vi "User Interface.vi"(8 "error in (no error)":errorcluster, 11 "User Interface in":refnum<class "User Interface.lvclass">) -> (0 "error out":errorcluster, 3 "User Interface out":refnum<class "User Interface.lvclass">)   [LabVIEW 2017, in "DSF Core.lvlib" / "Core Channel User Interface.lvclass"]
uses:
  Core Channel User Interface.lvclass
  User Interface.lvclass
  Configuration/Configuration.lvclass
  Configuration/Base/Channel/Channel Configuration.lvclass
  C:/Git/DSF/Core/Classes/Configuration/Configuration.lvclass
panel:
  out "Data Version":string
  in  "String Data Type":T1(ring)
  in  "Engine Data Type":T1(ring)
  in  "String Offset":u64 format="%d bytes"
  in  "Units":string
  in  "Name":string
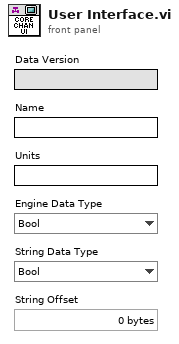
[diagram p1: front panel]
types:
  T1 = enum8{"Bool", "SGL", "DBL", "I8", "I16", "I32", "I64", "U8", "U16", "U32", "U64"}
  T2 = typedef "DSF Core.lvlib/DSF Core Channel Configuration.ctl" = cluster{"name":string, "units":string, "engine data type":T3, "string data type":T3, "string offset":u64}
  T3 = typedef "DSF Core.lvlib/DSF Data Type.ctl" = enum8{"Bool", "SGL", "DBL", "I8", "I16", "I32", "I64", "U8", "U16", "U32", "U64"}
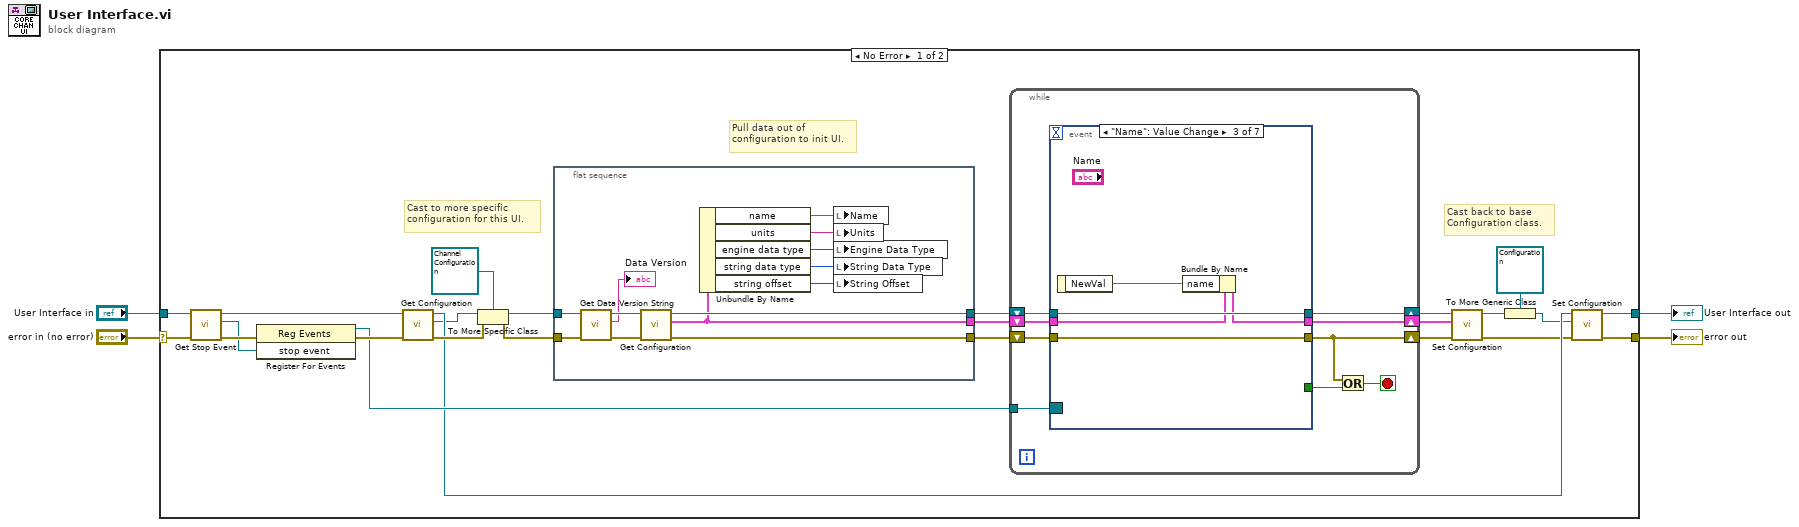
[diagram p0: block diagram]
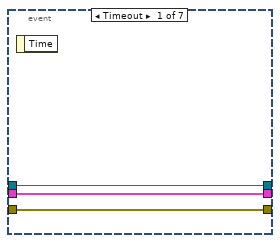
[diagram p2: hidden frame]
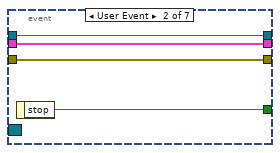
[diagram p3: hidden frame]
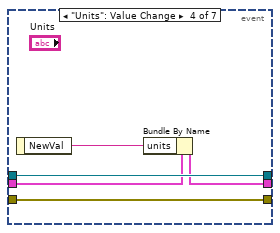
[diagram p4: hidden frame]
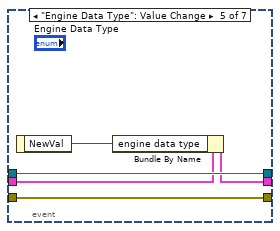
[diagram p5: hidden frame]
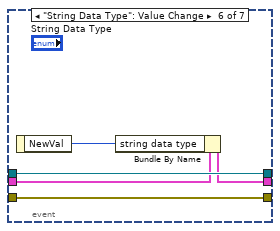
[diagram p6: hidden frame]
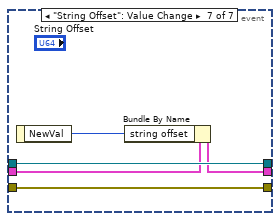
[diagram p7: hidden frame]
diagram:
  n1 = case shown="No Error" "error in (no error)" {
    selector: "error in (no error)" -> [w21 w85]
    tunnel: "User Interface in" -> [w20 w84]
    tunnel: [w14 w84] -> w1
    tunnel: [w15 w85] -> w3
    frame No Error {
      # "Pull data out of configuration to init UI."
      # "Cast back to base Configuration class."
      # "Cast to more specific configuration for this UI."
      n2 = call "Get Stop Event.vi"("error in (no error)"=w21, "User Interface in"=w20) -> ("error out"=w19:errorcluster, "stop event"=w18:refnum<user-event>, "User Interface out"=w17:refnum<class "User Interface.lvclass">)  [unwired: 7 in]
      n3 = register-events(error in=w19, w18) -> (reference out=w16:refnum<event-registration>, error out=w23:errorcluster)  [unwired: 1 in]
      n4 = call "Get Configuration.vi"("error in (no error)"=w23, "User Interface in"=w17) -> ("error out"=w22:errorcluster, "configuration"=w12:refnum<class "Configuration.lvclass">, "User Interface out"=w13:refnum<class "User Interface.lvclass">)  [unwired: 7 in]
      n5 = To More Specific Class(target class=refnum<class "Channel Configuration.lvclass"> refnum ("DSF Core.lvlib:Channel Configuration.lvclass"), reference=w12, error in=w22) -> (specific class reference=w27:refnum<class "Channel Configuration.lvclass">, error out=w28:errorcluster)
      n6 = flat-sequence {
        tunnel: [w32] -> w25
        tunnel: w28 -> [w36]
        tunnel: w27 -> [w37]
        tunnel: [w33] -> w26
        tunnel: [w31] -> w24
        frame #0 {
          n7 = call "Get Data Version String.vi"("error in (no error)"=w36, "Configuration in"=w37) -> ("error out"=w34:errorcluster, "data version"=→"Data Version":string, "Configuration out"=w35:refnum<class "Channel Configuration.lvclass">)  [unwired: 7 in]
          n8 = call "Get Configuration.vi"("error in (no error)"=w34, "Core Channel Configuration in"=w35) -> ("error out"=w32:errorcluster, "configuration"=w31:T2, "Core Channel Configuration out"=w33:refnum<class "Channel Configuration.lvclass">)  [unwired: 7 in]
          n9 = Unbundle By Name(w31) -> ("name"=w42:string, "units"=w41:string, "engine data type"=w40:T3, "string data type"=w39:T3, "string offset"=w38:u64)
          n10 = local write "Name"(w42) -> ()
          n11 = local write "Units"(w41) -> ()
          n12 = local write "Engine Data Type"(w40) -> ()
          n13 = local write "String Data Type"(w39) -> ()
          n14 = local write "String Offset"(w38) -> ()
        }
      }
      n15 = while {
        tunnel: w16 -> [w51]
        shift-right: [w49] -> w9
        shift-left: w25 -> [w50]
        shift-right: [w45] -> w7
        shift-left: w26 -> [w46]
        shift-right: [w43] -> w5
        shift-left: w24 -> [w44]
        stop <- w48 stop-if-true
        n16 = event shown="[2] \"Name\": Value Change" {
          selector: w51 -> [_ _ _ _ _ _ _]
          dyn-events: _ -> [_ _ _ _ _ _ _]
          timeout: _ -> [_ _ _ _ _ _ _]
          tunnel: [_ w56 _ _ _ _ _] -> w47
          tunnel: w50 -> [w54 w58 w62 w67 w72 w77 w82]
          tunnel: [w54 w58 w62 w67 w72 w77 w82] -> w49
          tunnel: w46 -> [w53 w57 w63 w68 w73 w78 w83]
          tunnel: [w53 w57 w63 w68 w73 w78 w83] -> w45
          tunnel: w44 -> [w52 w55 w60 w65 w70 w75 w80]
          tunnel: [w52 w55 w59 w64 w69 w74 w79] -> w43
          event Timeout {
            n17 = event-data() -> ()  [unwired: 1 in, 1 out]
          }
          event User Event {
            n18 = event-data() -> ("stop"=w56:bool)  [unwired: 1 in]
          }
          event "Name": Value Change {
            n19 = event-data() -> ("NewVal"=w61:string)  [unwired: 1 in]
            n20 = Bundle By Name(cluster=w60, "name"=w61) -> (w59:T2)
          }
          event "Units": Value Change {
            n21 = event-data() -> ("NewVal"=w66:string)  [unwired: 1 in]
            n22 = Bundle By Name(cluster=w65, "units"=w66) -> (w64:T2)
          }
          event "Engine Data Type": Value Change {
            n23 = event-data() -> ("NewVal"=w71:T1)  [unwired: 1 in]
            n24 = Bundle By Name(cluster=w70, "engine data type"=w71) -> (w69:T2)
          }
          event "String Data Type": Value Change {
            n25 = event-data() -> ("NewVal"=w76:T1)  [unwired: 1 in]
            n26 = Bundle By Name(cluster=w75, "string data type"=w76) -> (w74:T2)
          }
          event "String Offset": Value Change {
            n27 = event-data() -> ("NewVal"=w81:u64)  [unwired: 1 in]
            n28 = Bundle By Name(cluster=w80, "string offset"=w81) -> (w79:T2)
          }
        }
        n29 = Or(x=w49, y=w47) -> (x .or. y?=w48:bool)
      }
      n30 = call "Set Configuration.vi"("error in (no error)"=w9, "configuration"=w5, "Core Channel Configuration in"=w7) -> ("error out"=w8:errorcluster, "Core Channel Configuration out"=w6:refnum<class "Channel Configuration.lvclass">)  [unwired: 7 in]
      n31 = To More Generic Class(target class=refnum<class "Configuration.lvclass"> refnum ("Configuration out"), reference=w6) -> (generic class reference=w11:refnum<class "Configuration.lvclass">)
      n32 = call "Set Configuration.vi"("error in (no error)"=w8, "configuration"=w11, "User Interface in"=w13) -> ("error out"=w15:errorcluster, "User Interface out"=w14:refnum<class "User Interface.lvclass">)  [unwired: 7 in]
    }
    frame Error {
    }
  }
  "error out" <- w3
  "User Interface out" <- w1
